vi "String to Boolean_csm.vi"(1 "Default(F)":bool, 3 "String":string) -> (0 "Boolean":bool)   [LabVIEW 2017, in "API String Arguments Support.lvlib"]
doc: "If the input string is one of \"1\", \"Active\", \"Affirmed\", \"Enable\", \"Established\", \"Existing\", \"Non-null\", \"On\", \"operational\", \"T\", \"True\", \"valid\" , the output will be ture; if the input string is one of \"0\", \"Abolished\", \"Close\", \"Disable\", \"F\", \"False\", \"Inactive\", \"Inoperative\", \"Invalid\", \"Locked\", \"Negated\", \"Nonexistent\", \"Off\", \"void\" , the output will be false; otherwise, the outputs follows the default boolean control."
uses:
  API String Arguments Support.lvlib
  <userlib>/_NEVSTOP/Communicable State Machine(CSM)/Communicable State Machine.lvlib
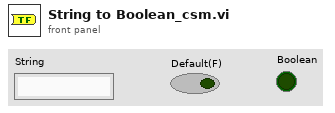
[diagram p1: front panel]
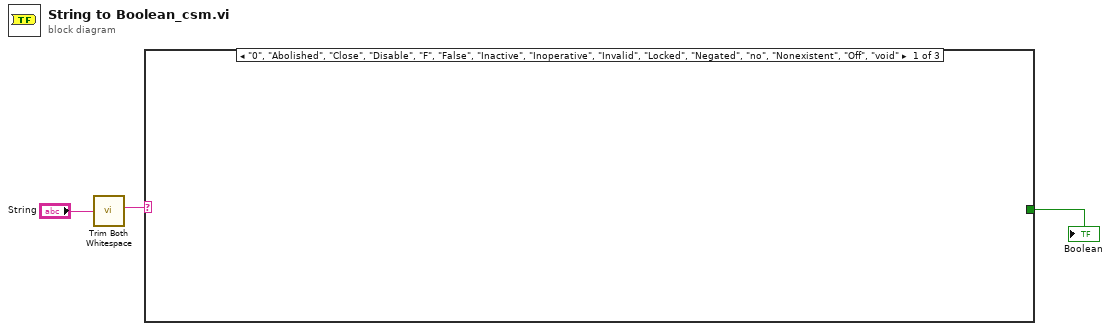
[diagram p0: block diagram]
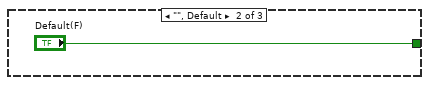
[diagram p2: hidden frame]
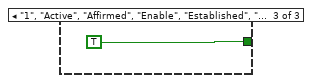
[diagram p3: hidden frame]
diagram:
  n1 = call <userlib>:"Trim Both Whitespace.vi"("string"="String") -> ("trimmed string"=w1:string)  [unwired: 1 in]
  n2 = case shown="\"0\", \"Abolished\", \"Close\", \"Disable\", \"F\", \"False\", \"Inactive\", \"Inoperative\", \"Invalid\", \"Locked\", \"Negated\", \"no\", \"Nonexistent\", \"Off\", \"void\"" w1 {
    tunnel: [_ "Default(F)" TRUE] -> w2
    frame "0", "Abolished", "Close", "Disable", "F", "False", "Inactive", "Inoperative", "Invalid", "Locked", "Negated", "no", "Nonexistent", "Off", "void" {
    }
    frame "", Default {
    }
    frame "1", "Active", "Affirmed", "Enable", "Established", "Existing", "Non-null", "On", "operational", "T", "True", "valid", "yes" {
    }
  }
  "Boolean" <- w2
